vi "PositionTorqueCurrentFOC Setter.vi"(0 "DeviceReference":T1, 3 "Update Frequency (Hz)":dbl=100.0, 5 "Position":dbl, 7 "FeedForward":dbl, 9 "Slot":i32) -> (4 "DeviceReference Out":T1)   [LabVIEW 2020]
doc: "Request PID to target position with duty-cycle feed forward.\nThis control mode will set the motor's position setpoint to the position specified by the user. In addition, it will apply an additional torque current as an arbitrary feed-forward value."
uses:
  DeviceReference.ctl
  <userlib>/CTRE_PhoenixTools/CTRE_PhoenixTools.lvlib
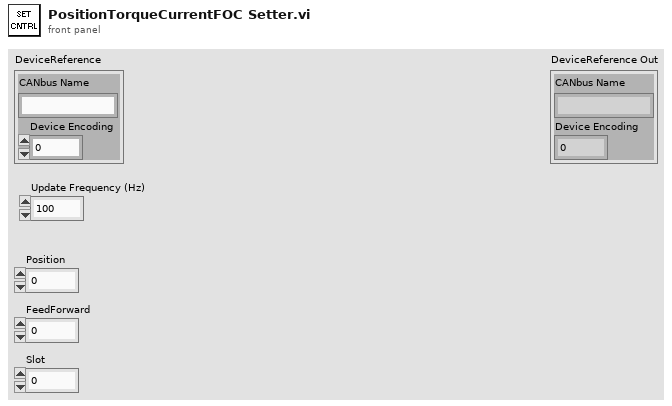
[diagram p1: front panel]
types:
  T1 = typedef "DeviceReference.ctl" = cluster{"CANbus Name":string, "Device Encoding":u32}
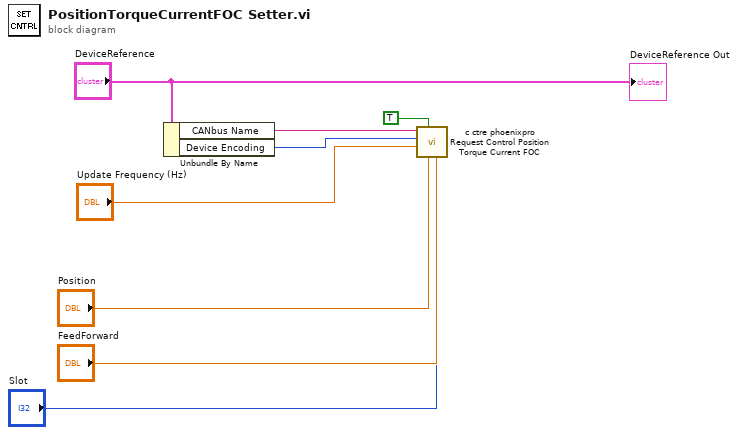
[diagram p0: block diagram]
diagram:
  n1 = Unbundle By Name("DeviceReference") -> ("CANbus Name"=w7:string, "Device Encoding"=w6:u32)
  n2 = call <userlib>:"c ctre phoenixpro Request Control Position Torque Current FOC.vi"("Slot"="Slot", "FeedForward"="FeedForward", "Position"="Position", "cancelOtherRequests"=TRUE, "updateTime"="Update Frequency (Hz)", "ecuEncoding"=w6, "canbus"=w7) -> ()  [unwired: 3 in, 2 out]
  "DeviceReference Out" <- "DeviceReference"
